vi "Pose3DtoVector3D.vi"(9 "Tail":T2, 11 "Nose":T2) -> (3 "Vector3D":T1)   [LabVIEW 2018]
uses:
  Pose3D.ctl
  Vector/Vector3D.ctl
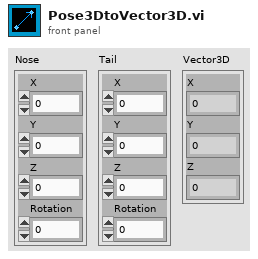
[diagram p1: front panel]
types:
  T1 = typedef "Vector3D.ctl" = cluster{"X":dbl, "Y":dbl, "Z":dbl}
  T2 = typedef "Pose3D.ctl" = cluster{"X":dbl, "Y":dbl, "Z":dbl, "Rotation":dbl}
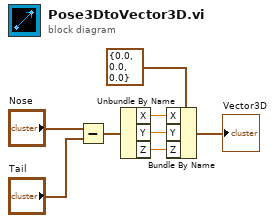
[diagram p0: block diagram]
diagram:
  n1 = Subtract(x="Nose", y="Tail") -> (x-y=w6:T2)
  n2 = Unbundle By Name(w6) -> ("X"=w4:dbl, "Y"=w3:dbl, "Z"=w1:dbl)
  n3 = Bundle By Name(cluster=T1 {"X"=0.0, "Y"=0.0, "Z"=0.0} ("Vector 2"), "X"=w4, "Y"=w3, "Z"=w1) -> (→"Vector3D":T1)
